vi "armEncoderCountsToAngle.vi"(1 "armEncoderCount":dbl) -> (0 "armAngle":dbl)   [LabVIEW 2020]
panel:
  in  "b":dbl=6.3008
  in  "m":dbl=0.50267
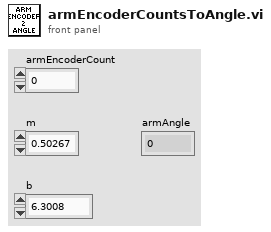
[diagram p1: front panel]
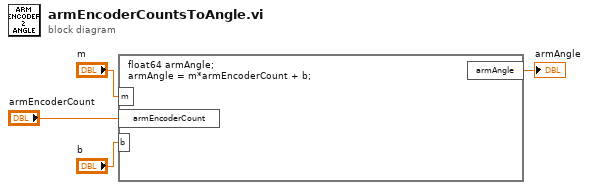
[diagram p0: block diagram]
diagram:
  n1 = formula code="float64 armAngle;\narmAngle = m*armEncoderCount + b;"("m"="m", "armEncoderCount"="armEncoderCount", "b"="b") -> ("armAngle"=→"armAngle":dbl)
